vi "Pre Launch Init.vi"(11 "UI Actor in":refnum<class "UI Actor.lvclass">) -> (0 "error out":errorcluster, 3 "UI Actor out":refnum<class "UI Actor.lvclass">)   [LabVIEW 2024, in "UI Actor.lvlib" / "UI Actor.lvclass"]
doc: "Initializes the panel actor. Creates the Panel Helper.\n\n----\nPlease see the following web address for additional documentation and tutorial information:\nhttp://www.mooregoodideas.com/mgi-panel-manager/\n\nAuthor: Derek Trepanier\n\nCopyright (c) 2018, Moore Good Ideas, Inc.\n\nAll rights reserved.\n\nRedistribution and use in source and binary forms, with or without modification, are permitted provided that the following conditions are met:\n\n * Redistributions of source code must retain the above copyright notice, this list of conditions and the following disclaimer.\n * Redistributions in binary form must reproduce the above copyright notice, this list of conditions and the following disclaimer in the documentation and/or other materials provided with the distribution.\n * Neither the name of Moore Good Ideas, Inc. nor the names of its contributors may be used to endorse or promote products derived from this software without specific prior written permission.\n\nTHIS SOFTWARE IS PROVIDED BY THE COPYRIGHT HOLDERS AND CONTRIBUTORS \"AS IS\" AND ANY EXPRESS OR IMPLIED WARRANTIES, INCLUDING, BUT NOT LIMITED TO, THE IMPLIED WARRANTIES OF MERCHANTABILITY AND FITNESS FOR A PARTICULAR PURPOSE ARE DISCLAIMED. IN NO EVENT SHALL THE COPYRIGHT OWNER OR CONTRIBUTORS BE LIABLE FOR ANY DIRECT, INDIRECT, INCIDENTAL, SPECIAL, EXEMPLARY, OR CONSEQUENTIAL DAMAGES (INCLUDING, BUT NOT LIMITED TO, PROCUREMENT OF SUBSTITUTE GOODS OR SERVICES; LOSS OF USE, DATA, OR PROFITS; OR BUSINESS INTERRUPTION) HOWEVER CAUSED AND ON ANY THEORY OF LIABILITY, WHETHER IN CONTRACT, STRICT LIABILITY, OR TORT (INCLUDING NEGLIGENCE OR OTHERWISE) ARISING IN ANY WAY OUT OF THE USE OF THIS SOFTWARE, EVEN IF ADVISED OF THE POSSIBILITY OF SUCH DAMAGE."
uses:
  UI Actor.lvclass
  Controls/Supported Baudrates.ctl
  Controls/Device Info.ctl
  Controls/File Info.ctl
  Controls/Device Settings.ctl
  UI Actor.lvclass/UI Actor.ctl
  <vilib>/MGI/Panel Manager/Panel Actor/Panel Actor/Panel Actor.lvclass
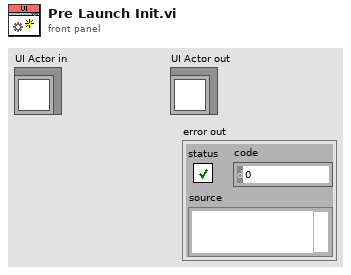
[diagram p1: front panel]
types:
  T1 = typedef "Device Settings.ctl" = cluster{"SimpleBootUpSlave":bool, "SimpleBootUpMaster":bool}
  T2 = typedef "File Info.ctl" = cluster{"FileVersion":string, "FileRevision":u8, "EDSVersion":string, "Description":string, "CreationDate":string, "CreationTime":string, "CreatedBy":string, "ModificationDate":string, "ModificationTime":string, "ModifiedBy":string}
  T3 = typedef "Device Info.ctl" = cluster{"ProductName":string, "ProductNumber":string, "VendorName":string, "VendorNumber":string}
  T4 = typedef "Supported Baudrates.ctl" = cluster{"BaudRate_10":bool, "BaudRate_20":bool, "BaudRate_50":bool, "BaudRate_125":bool, "BaudRate_250":bool, "BaudRate_500":bool, "BaudRate_800":bool, "BaudRate_1000":bool, "BaudRate_auto":bool}
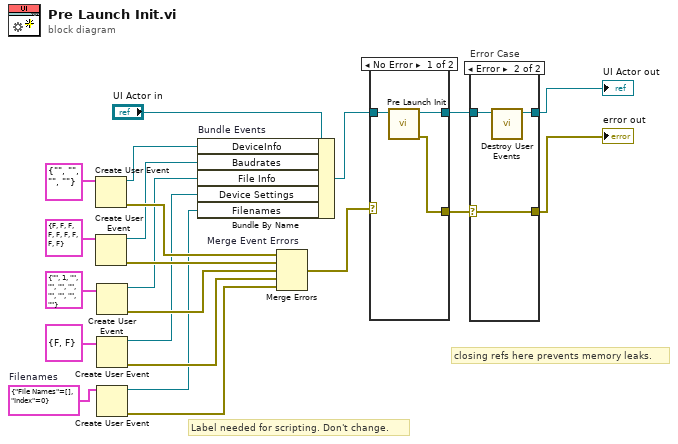
[diagram p0: block diagram]
diagram:
  w2 = cluster{"File Names":string[], "Index":i32} {"File Names"=[], "Index"=0}  # Filenames
  # "closing refs here prevents memory leaks."
  # "Label needed for scripting. Don't change."
  n1 = Create User Event(user event datatype=T3 {"ProductName"="", "ProductNumber"="", "VendorName"="", "VendorNumber"=""} ("DeviceInfo")) -> (user event=w14:refnum<user-event>, error out=w16:errorcluster)  [unwired: 1 in]
  n2 = Create User Event(user event datatype=T4 {"BaudRate_10"=FALSE, "BaudRate_20"=FALSE, "BaudRate_50"=FALSE, "BaudRate_125"=FALSE, "BaudRate_250"=FALSE, "BaudRate_500"=FALSE, "BaudRate_800"=FALSE, "BaudRate_1000"=FALSE, "BaudRate_auto"=FALSE} ("Baudrates")) -> (user event=w10:refnum<user-event>, error out=w11:errorcluster)  [unwired: 1 in]
  n3 = Create User Event(user event datatype=T2 {"FileVersion"="", "FileRevision"=1, "EDSVersion"="", "Description"="", "CreationDate"="", "CreationTime"="", "CreatedBy"="", "ModificationDate"="", "ModificationTime"="", "ModifiedBy"=""} ("EDS File Info")) -> (user event=w7:refnum<user-event>, error out=w8:errorcluster)  [unwired: 1 in]
  n4 = Create User Event(user event datatype=T1 {"SimpleBootUpSlave"=FALSE, "SimpleBootUpMaster"=FALSE} ("Device Settings")) -> (user event=w5:refnum<user-event>, error out=w4:errorcluster)  [unwired: 1 in]
  n5 = Create User Event(user event datatype=w2) -> (user event=w1:refnum<user-event>, error out=w3:errorcluster)  [unwired: 1 in]
  n6 = Bundle By Name "Bundle Events"(cluster="UI Actor in", "DeviceInfo"=w14, "Baudrates"=w10, "File Info"=w7, "Device Settings"=w5, "Filenames"=w1) -> (w17:refnum<class "UI Actor.lvclass">)
  n7 = Merge Errors "Merge Event Errors"(w16, w11, w8, w4, w3) -> (w15:errorcluster)
  n8 = case shown="No Error" w15 {
    selector: w15 -> [_ w26]
    tunnel: w17 -> [w25 w27]
    tunnel: [w24 w27] -> w22
    tunnel: [w23 w26] -> w20
    frame No Error {
      n9 = call-parent "Pre Launch Init.vi"("Panel Actor in"=w25) -> ("error out"=w23:errorcluster, "Panel Actor out"=w24:refnum<class "UI Actor.lvclass">)  [unwired: 9 in]
    }
    frame Error {
    }
  }
  n10 = case "Error Case" shown="Error" w20 {
    selector: w20 -> [w28 w32]
    tunnel: w22 -> [w29 w31]
    tunnel: [w29 w30] -> w21
    tunnel: [w28 w32] -> w19
    frame No Error {
    }
    frame Error {
      n11 = call "Destroy User Events.vi"("UI Actor in"=w31) -> ("UI Actor out"=w30:refnum<class "UI Actor.lvclass">)  [unwired: 10 in]
    }
  }
  "error out" <- w19
  "UI Actor out" <- w21
